vi "Initialize Menu Items.vi"(8 "error in (no error)":errorcluster, 10 "Config":T1, 11 "Menu Ref":refnum<k9>) -> (0 "error out":errorcluster)   [LabVIEW 2023, in "VI Properties Editor.lvlib"]
doc: "Initializes several menu items related to options and recently viewed folders/files in <B>Config</B>."
uses:
  VI Properties Editor.lvlib
  CTLs/Config.ctl
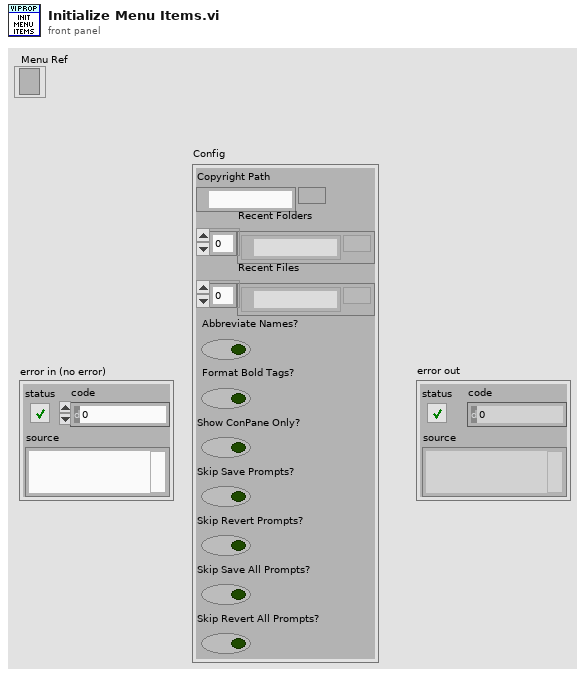
[diagram p1: front panel]
types:
  T1 = typedef "VI Properties Editor.lvlib/Config.ctl" = cluster{"Copyright Path":path, "Recent Folders":path[], "Recent Files":path[], "Abbreviate Names?":bool, "Format Bold Tags?":bool, "Show ConPane Only?":bool, "Skip Save Prompts?":bool, "Skip Revert Prompts?":bool, "Skip Save All Prompts?":bool, "Skip Revert All Prompts?":bool}
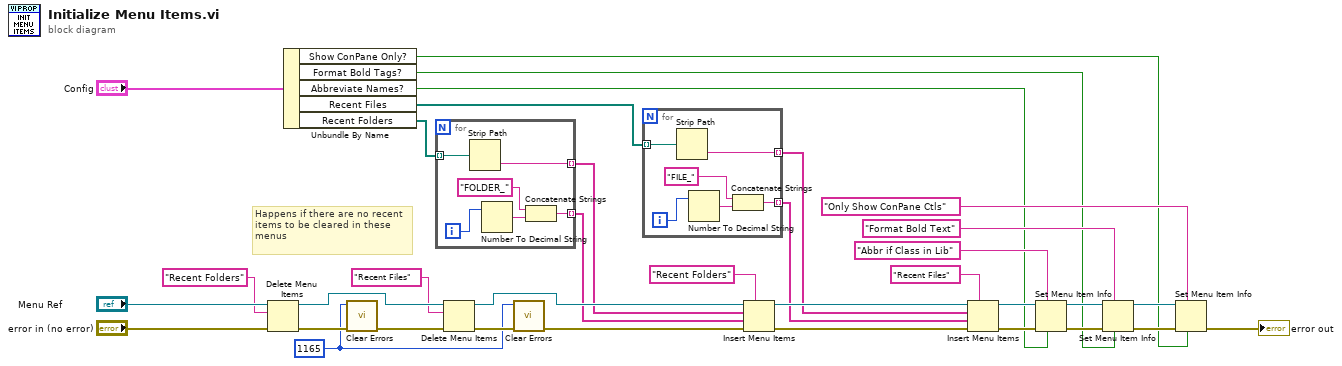
[diagram p0: block diagram]
diagram:
  w4 = 1165
  # "Happens if there are no recent items to be cleared in these menus"
  n1 = Delete Menu Items(6:"error in (no error)", 8:"Recent Folders" ("menu tag"), 9:"Menu Ref") -> (0:w10:errorcluster, 3:w34:refnum<k9>)  [unwired: 1 in]
  n2 = Unbundle By Name("Config") -> ("Show ConPane Only?"=w1:bool, "Format Bold Tags?"=w12:bool, "Abbreviate Names?"=w13:bool, "Recent Files"=w16:path[], "Recent Folders"=w23:path[])
  n3 = call <vilib>:"Clear Errors.vi"("error in (no error)"=w10, "specific error code to clear (0: all)"=w4) -> ("error out"=w5:errorcluster)  [unwired: 4 in, 1 out]
  n4 = for {
    tunnel: w23 -> [w40] mode=indexing
    tunnel: [w37] -> w17 mode=indexing
    tunnel: [w36] -> w18 mode=indexing
    i -> [w41]
    n5 = Strip Path(path=w40) -> (name=w36:string)  [unwired: 1 out]
    n6 = Number To Decimal String(number=w41) -> (decimal integer string=w39:string)  [unwired: 1 in]
    n7 = Concatenate Strings("FOLDER_", w39) -> (w37:string)
  }
  n8 = Delete Menu Items(6:w5, 8:"Recent Files" ("menu tag"), 9:w34) -> (0:w11:errorcluster, 3:w33:refnum<k9>)  [unwired: 1 in]
  n9 = call <vilib>:"Clear Errors.vi"("error in (no error)"=w11, "specific error code to clear (0: all)"=w4) -> ("error out"=w6:errorcluster)  [unwired: 4 in, 1 out]
  n10 = for {
    tunnel: w16 -> [w46] mode=indexing
    tunnel: [w43] -> w15 mode=indexing
    tunnel: [w42] -> w14 mode=indexing
    i -> [w47]
    n11 = Strip Path(path=w46) -> (name=w42:string)  [unwired: 1 out]
    n12 = Number To Decimal String(number=w47) -> (decimal integer string=w45:string)  [unwired: 1 in]
    n13 = Concatenate Strings("FILE_", w45) -> (w43:string)
  }
  n14 = Insert Menu Items(5:"Recent Folders" ("menu tag"), 6:w6, 7:w17, 8:w18, 9:w33) -> (0:w29:errorcluster, 3:w20:refnum<k9>)  [unwired: 1 in, 1 out]
  n15 = Insert Menu Items(5:"Recent Files" ("menu tag"), 6:w29, 7:w15, 8:w14, 9:w20) -> (0:w28:errorcluster, 3:w19:refnum<k9>)  [unwired: 1 in, 1 out]
  n16 = Set Menu Item Info(6:w13, 7:"Abbr if Class in Lib" ("menu tag"), 8:w28, 11:w19) -> (0:w32:errorcluster, 3:w25:refnum<k9>)  [unwired: 3 in]
  n17 = Set Menu Item Info(6:w12, 7:"Format Bold Text" ("item tag"), 8:w32, 11:w25) -> (0:w31:errorcluster, 3:w2:refnum<k9>)  [unwired: 3 in]
  n18 = Set Menu Item Info(6:w1, 7:"Only Show ConPane Ctls" ("item tag"), 8:w31, 11:w2) -> (0:→"error out":errorcluster)  [unwired: 3 in, 1 out]
